vi "FGV_PSP - IPS120 Status.vi"(4 "error in":errorcluster, 6 "Function":enum16{"write", "read"}(ring), 7 "status":T1) -> (0 "error out":errorcluster, 3 "status":T1)   [LabVIEW 2013]
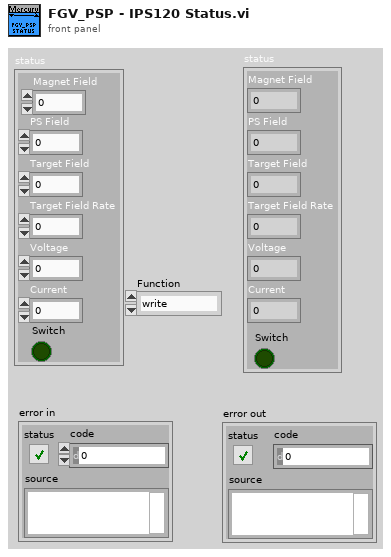
[diagram p1: front panel]
types:
  T1 = cluster{"Magnet Field":dbl, "PS Field":dbl, "Target Field":dbl, "Target Field Rate":dbl, "Voltage":dbl, "Current":dbl, "Switch":bool}
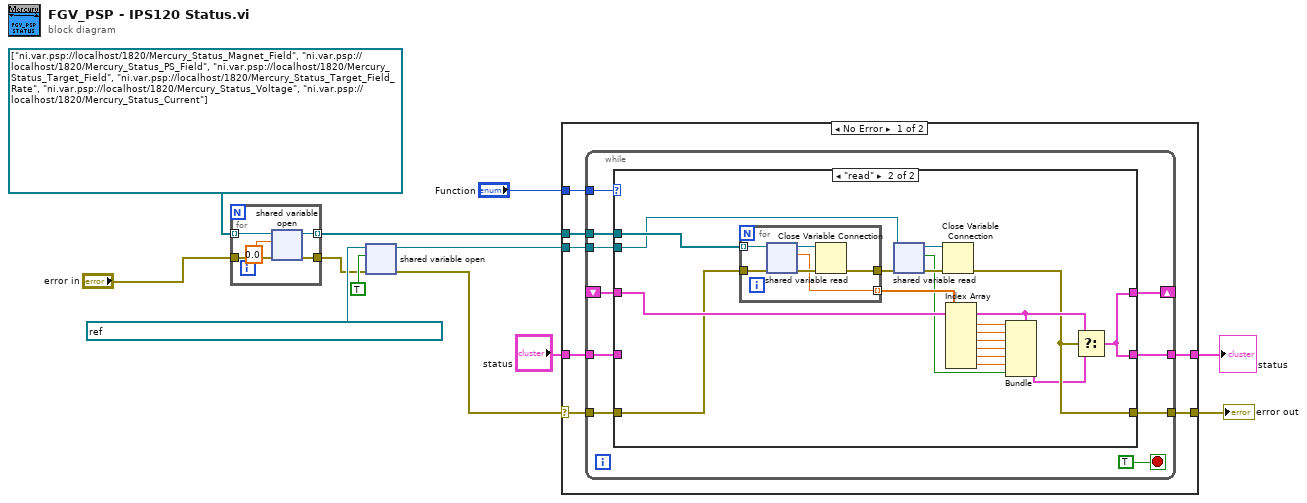
[diagram p0: block diagram]
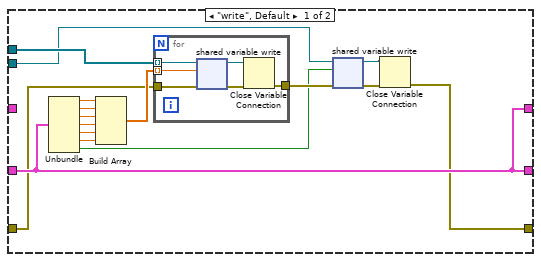
[diagram p2: hidden frame]
diagram:
  n1 = for {
    tunnel: refnum<k21>[] ["ni.var.psp://localhost/1820/Mercury_Status_Magnet_Field", "ni.var.psp://localhost/1820/Mercury_Status_PS_Field", "ni.var.psp://localhost/1820/Mercury_Status_Target_Field", "ni.var.psp://localhost/1820/Mercury_Status_Target_Field_Rate", "ni.var.psp://localhost/1820/Mercury_Status_Voltage", "ni.var.psp://localhost/1820/Mercury_Status_Current"] -> [w17] mode=indexing
    tunnel: [w15] -> w3 mode=indexing
    tunnel: [w14] -> w5
    tunnel: "error in" -> [w13]
    n2 = shared-variable-open(w17, w13, 0.0) -> (w15:refnum<k21>, w14:errorcluster)  [unwired: 1 in]
  }
  n3 = shared-variable-open(refnum<k21> "ni.var.psp://localhost/1820/Mercury_Status_Switch" ("shared variable refnum in"), w5, TRUE) -> (w2:refnum<k21>, w1:errorcluster)  [unwired: 1 in]
  n4 = case shown="No Error" w1 {
    selector: w1 -> [w24 w82]
    tunnel: [w23 w82] -> w12
    tunnel: "status" -> [w22 w81]
    tunnel: [w21 w81] -> w9
    tunnel: "Function" -> [w20 _]
    tunnel: w3 -> [w19 _]
    tunnel: w2 -> [w18 _]
    frame No Error {
      n5 = while {
        shift-right: [w28] -> _
        shift-left: _ -> [w27]
        tunnel: w24 -> [w33]
        tunnel: [w32] -> w23
        tunnel: w22 -> [w31]
        tunnel: [w30] -> w21
        tunnel: w20 -> [w29]
        tunnel: w19 -> [w26]
        tunnel: w18 -> [w25]
        stop <- TRUE stop-if-true
        n6 = case shown="\"read\"" w29 {
          tunnel: w33 -> [w38 w61]
          tunnel: [w37 w60] -> w32
          tunnel: w31 -> [w50 _]
          tunnel: [w50 w63] -> w30
          tunnel: [w50 w63] -> w28
          tunnel: w27 -> [_ w64]
          tunnel: w26 -> [w43 w74]
          tunnel: w25 -> [w36 w59]
          frame "write", Default {
            n7 = Unbundle(w50) -> ("Magnet Field"=w49:dbl, "PS Field"=w44:dbl, "Target Field"=w45:dbl, "Target Field Rate"=w46:dbl, "Voltage"=w47:dbl, "Current"=w48:dbl, "Switch"=w39:bool)
            n8 = Build Array(w49, w44, w45, w46, w47, w48) -> (w42:dbl[])
            n9 = for {
              tunnel: w38 -> [w56]
              tunnel: w43 -> [w53] mode=indexing
              tunnel: w42 -> [w52] mode=indexing
              tunnel: [w51] -> w40
              n10 = shared-variable-write(w53, w56, w52) -> (w54:refnum<k21>, w55:errorcluster)
              n11 = Close Variable Connection(8:w55, 11:w54) -> (0:w51:errorcluster)
            }
            n12 = shared-variable-write(w36, w40, w39) -> (w35:refnum<k21>, w41:errorcluster)
            n13 = Close Variable Connection(8:w41, 11:w35) -> (0:w37:errorcluster)
          }
          frame "read" {
            n14 = for {
              tunnel: w74 -> [w80] mode=indexing
              tunnel: [w76] -> w62 mode=indexing
              tunnel: [w77] -> w66
              tunnel: w61 -> [w75]
              n15 = shared-variable-read(w80, w75) -> (w79:refnum<k21>, w78:errorcluster, w76:dbl)  [unwired: 1 out]
              n16 = Close Variable Connection(8:w78, 11:w79) -> (0:w77:errorcluster)
            }
            n17 = shared-variable-read(w59, w66) -> (w67:refnum<k21>, w65:errorcluster, w58:bool)  [unwired: 1 out]
            n18 = Close Variable Connection(8:w65, 11:w67) -> (0:w60:errorcluster)
            n19 = Index Array(array=w62) -> (element #1=w73:dbl, element #2=w68:dbl, element #3=w69:dbl, element #4=w70:dbl, element #5=w71:dbl, element #6=w72:dbl)  [unwired: 6 in]
            n20 = Bundle(cluster=w64, "Magnet Field"=w73, "PS Field"=w68, "Target Field"=w69, "Target Field Rate"=w70, "Voltage"=w71, "Current"=w72, "Switch"=w58) -> (w57:T1)
            n21 = Select(t=w64, s=w60, f=w57) -> (s? t:f=w63:T1)
          }
        }
      }
    }
    frame Error {
    }
  }
  "error out" <- w12
  "status" <- w9
